vi "Init.vi"(8 "error in (no error)":errorcluster, 11 "Profile Name":string) -> (0 "error out":errorcluster, 3 "SetCurrentProfile out":refnum<class "RemoveProfile.lvclass">)   [LabVIEW 2020, in "obs-websocket.lvlib" / "RemoveProfile.lvclass"]
uses:
  RemoveProfile.lvclass
  RemoveProfile.lvclass/RemoveProfile.ctl
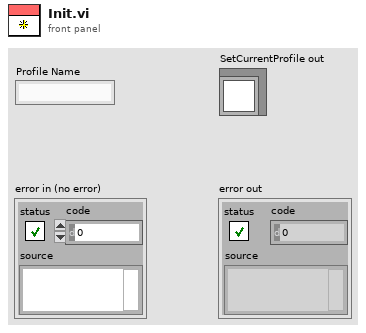
[diagram p1: front panel]
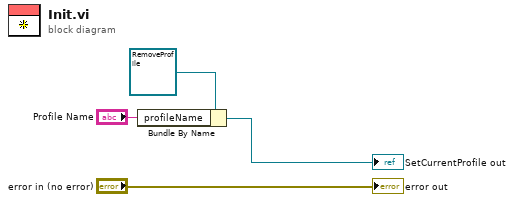
[diagram p0: block diagram]
diagram:
  n1 = Bundle By Name(cluster=refnum<class "RemoveProfile.lvclass"> refnum ("SetCurrentProfile in"), "profileName"="Profile Name") -> (→"SetCurrentProfile out":refnum<class "RemoveProfile.lvclass">)
  "error out" <- "error in (no error)"
